vi "hydraharp_parse_records.vi"(8 "error in (no error)":errorcluster, 11 "hydraharp in":refnum<class "hydraharp.lvclass">) -> (0 "error out":errorcluster, 3 "hydraharp out":refnum<class "hydraharp.lvclass">)   [LabVIEW 2015, in "hydraharp.lvclass"]
uses:
  hydraharp.lvclass
  hydraharp.lvclass/hydraharp.ctl
  hydraharp_panel/hpanel_acq_modes.ctl
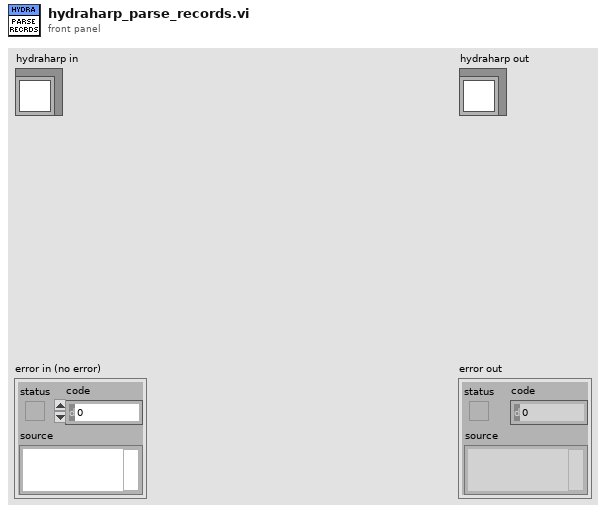
[diagram p1: front panel]
types:
  T1 = typedef "hpanel_acq_modes.ctl" = u16
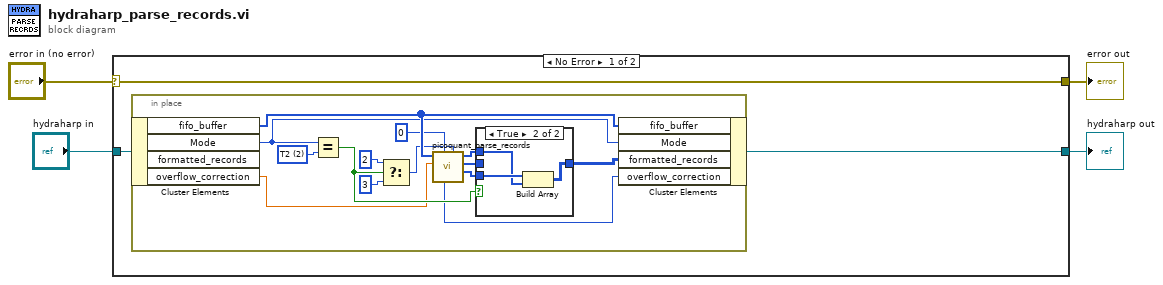
[diagram p0: block diagram]
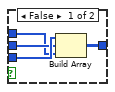
[diagram p2: hidden frame]
diagram:
  n1 = case shown="No Error" "error in (no error)" {
    selector: "error in (no error)" -> [w7 w30]
    tunnel: [w7 w30] -> w3
    tunnel: [w5 w29] -> w1
    tunnel: "hydraharp in" -> [w6 w29]
    frame No Error {
      n2 = in-place {
        w21 = T1 2 items=["T2"=2, "T3"=3] ("Mode")
        n3 = in-place-cluster #1(w6) -> ("fifo_buffer"=w15:u32[], "Mode"=w14:T1, "overflow_correction"=w10:dbl)  [unwired: 1 out]
        n4 = Equal?(x=w14, y=w21) -> (x = y?=w12:bool)
        n5 = Select(t=u8 2 ("tmode"), s=w12, f=u8 3) -> (s? t:f=w8:u8)
        n6 = call "picoquant_parse_records.vi"("acq_mode"=w8, "Device"=u8 0 ("device"), "overflow"=w10, "fifo_buffer"=w15) -> ("sync"=w18:u64[], "channels"=w17:u8[], "times"=w16:u64[], "overflow"=w9:u64)  [unwired: 2 in, 2 out]
        n7 = case shown="True" w12 {
          tunnel: w18 -> [w25 w28]
          tunnel: w17 -> [w24 _]
          tunnel: w16 -> [w23 w27]
          tunnel: [w22 w26] -> w13
          frame False {
            n8 = Build Array(w25, w24, w23) -> (w22:u64[][])
          }
          frame True {
            n9 = Build Array(w28, w27) -> (w26:u64[][])
          }
        }
        n10 = in-place-cluster #1("fifo_buffer"=w15, "Mode"=w14, "formatted_records"=w13, "overflow_correction"=w9) -> (w5:refnum<class "hydraharp.lvclass">)
      }
    }
    frame Error {
    }
  }
  "error out" <- w3
  "hydraharp out" <- w1
